vi "Convert Data to DTCs.vi"(7 "DTC descriptor":T2={"DTC Byte Length"=2, "Status Byte Length"=1, "Add Data Byte Length"=0, "Byte Order"=enum."Motorola"}, 8 "error in (no error)":errorcluster, 11 "All DTCs":T3[](array[typedef]) {"payload" format="%x"; "timestamp" format="%<%.7X\n%x>T"; "type" items=["CAN Data"=0, "CAN Remote"=1, "CAN Bus Error"=2, "J1939 Data"=192, "Delay"=224, "Log Trigger"=225, "Start Trigger"=226]; "identifier" format="%x"}) -> (0 "error out":errorcluster, 3 "DTCs":T1[](array[typedef]))   [LabVIEW 2015, in "GMLAN.lvlib"]
uses:
  GMLAN.lvlib
  <vilib>/xnet/xnet.llb/XNET Frame CAN.ctl
  <vilib>/xnet/xnet.llb/XNET Frame Type CAN.ctl
  <vilib>/Automotive Diagnostic Command Set/Diagnostic Protocols.llb/DTC Descriptor.ctl
  <vilib>/Automotive Diagnostic Command Set/Diagnostic Protocols.llb/Diagnostic Trouble Code.ctl
  <vilib>/Automotive Diagnostic Command Set/Diagnostic Protocols.llb/Convert to Phys.vi
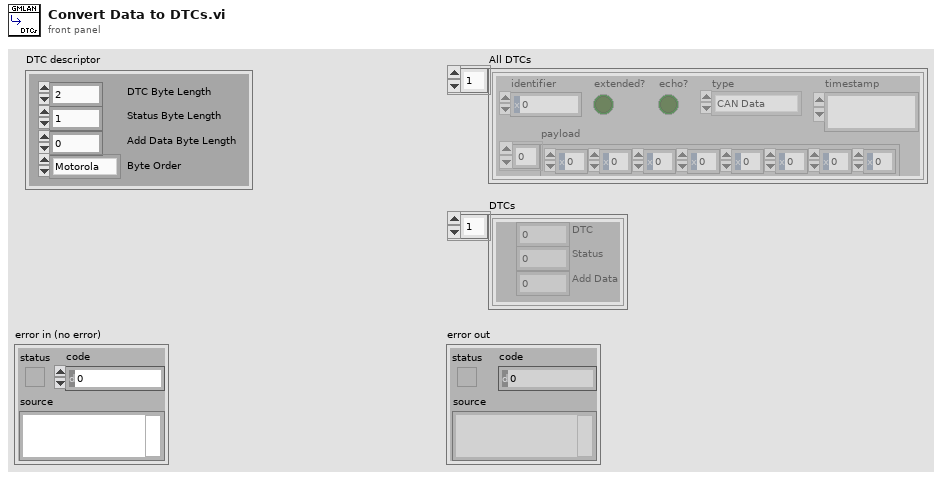
[diagram p1: front panel]
types:
  T1 = typedef "Diagnostic Trouble Code.ctl" = cluster{"DTC":u32, "Status":u32, "Add Data":u32}
  T2 = typedef "DTC Descriptor.ctl" = cluster{"DTC Byte Length":i32, "Status Byte Length":i32, "Add Data Byte Length":i32, "Byte Order":enum16{"Motorola", "Intel"}}
  T3 = typedef "XNET Frame CAN.ctl" = cluster{"timestamp":timestamp, "payload":u8[], "identifier":u32, "type":T4, "extended?":bool, "echo?":bool}
  T4 = typedef "XNET Frame Type CAN.ctl" = u8
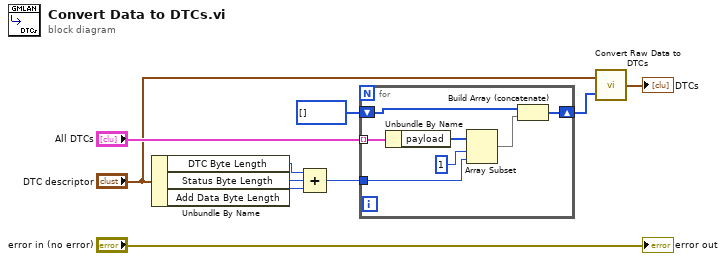
[diagram p0: block diagram]
diagram:
  n1 = Unbundle By Name("DTC descriptor") -> ("DTC Byte Length"=w8:i32, "Status Byte Length"=w7:i32, "Add Data Byte Length"=w5:i32)
  n2 = Compound Arithmetic op=ADD(w8, w7, w5) -> (w6:i32)
  n3 = for {
    tunnel: "All DTCs" -> [w17] mode=indexing
    shift-right: [w12] -> w3
    shift-left: u8[] [] -> [w14]
    tunnel: w6 -> [w11]
    n4 = Unbundle By Name(w17) -> ("payload"=w16:u8[])
    n5 = Array Subset(array=w16, index=1, length=w11) -> (w13:u8[])
    n6 = Build Array (concatenate)(w14, w13) -> (w12:u8[])
  }
  n7 = call "Convert Raw Data to DTCs.vi"("data in"=w3, "DTC descriptor"="DTC descriptor") -> ("DTCs"=→"DTCs":T1[])
  "error out" <- "error in (no error)"
